vi "Clear Cache.vi"   [LabVIEW 2016]
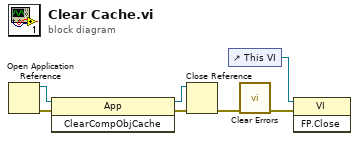
[diagram p0: block diagram]
diagram:
  n1 = Open Application Reference() -> (0:w4:errorcluster, 3:w7:refnum<vi>)  [unwired: 4 in]
  n2 = invoke class="App" method="ClearCompObjCache"(reference=w7, error in=w4) -> (reference out=w6:refnum<vi>, error out=w5:errorcluster)  [unwired: 1 in, 1 out]
  n3 = Close Reference(reference=w6, error in (no error)=w5) -> (error out=w3:errorcluster)
  n4 = control-ref of="This VI"() -> (w2:refnum<vi>)
  n5 = call <vilib>:"Clear Errors.vi"("error in (no error)"=w3) -> ("error out"=w1:errorcluster)  [unwired: 5 in, 1 out]
  n6 = invoke class="VI" method="FP.Close"(reference=w2, error in=w1) -> ()  [unwired: 1 in, 3 out]
